vi "Make Zoom String.vi"(8 "error in (no error)":errorcluster, 10 "Zoom (15)":u8 step=1) -> (0 "error out":errorcluster, 2 "Zoom string":string)   [LabVIEW 2012]
doc: "Creates the required zoom string."
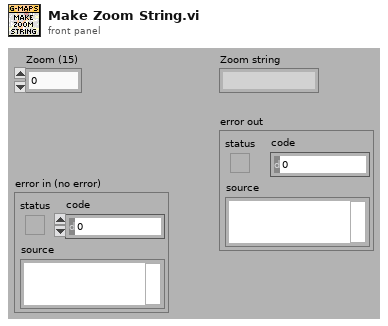
[diagram p1: front panel]
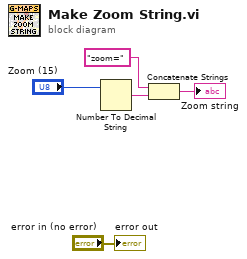
[diagram p0: block diagram]
diagram:
  n1 = Number To Decimal String(number="Zoom (15)") -> (decimal integer string=w1:string)  [unwired: 1 in]
  n2 = Concatenate Strings("zoom=" ("URL"), w1) -> (→"Zoom string":string)
  "error out" <- "error in (no error)"
